vi "FID Rohwerte Linearisieren.vi"(1 "GasValue":sgl[](array[numeric]), 12 "CAL-Daten":T1={"CH4 Null"=0.0, "CH4 Steil"=[1.0, 1.0, 1.0, 1.0], "THC Null"=0.0, "THC Steil"=[1.0, 1.0, 1.0, 1.0], "NMHC Null"=0.0, "NMHC Steil"=[1.0, 1.0, 1.0, 1.0]}) -> (4 "Messwerte":sgl[](array[numeric]), 6 "Rohwert":sgl[](array[numeric]), 8 "Rohwert LIN":sgl[](array[numeric]))   [LabVIEW 2020, in "ABB-EL3000.lvlib" / "FID.lvlib" / "FID Kalibrierung.lvlib"]
uses:
  FID Kalibrierung.lvlib
  Allgemeine VI/CAL-Daten FID.ctl
  Analysator Definition/FGV Analysator Definition Aktionen.ctl
  Analysator Definition/Analysator Definition.lvlib
  Linearisierung V2/Linearisierung v2.lvlib
  FID.lvlib
  Allgemeine VI/Allgemeine VI.lvlib
panel:
  in  "Rohwert umschalten":bool
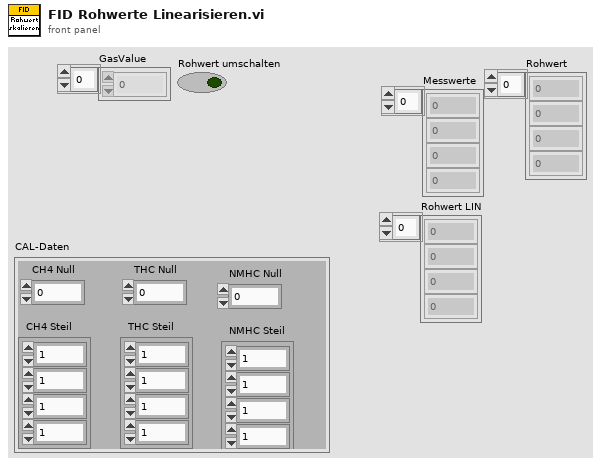
[diagram p1: front panel]
types:
  T1 = typedef "ABB-EL3000.lvlib/Allgemeine VI.lvlib/CAL-Daten FID.ctl" = cluster{"CH4 Null":sgl, "CH4 Steil":sgl[], "THC Null":sgl, "THC Steil":sgl[], "NMHC Null":sgl, "NMHC Steil":sgl[]}
  T2 = typedef "Analysator Definition.lvlib/FGV Analysator Definition Aktionen.ctl" = enum16{"lesen", "MB setzen", "MB KAL setzen", "laden"}
  T3 = typedef "Analysator Definition.lvlib/Betriebsdaten Komponente.ctl" = cluster{"Namen":string[], "MB Namen":string[], "Einheit":string, "MB Aktuell":u16, "MB Endwert":u16, "CalGase":u16[], "MB für KAL":u16[], "CG für KAL":u16[]}
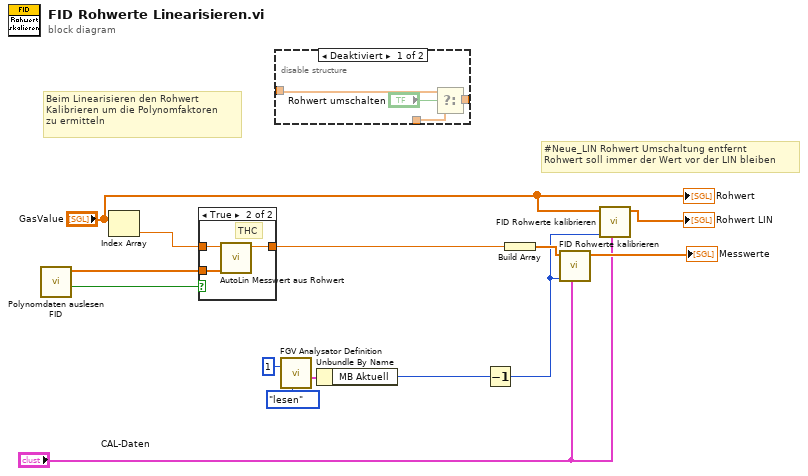
[diagram p0: block diagram]
diagram:
  # "#Neue_LIN Rohwert Umschaltung entfernt\nRohwert soll immer der Wert vor der LIN bleiben"
  # "Beim Linearisieren den Rohwert \nKalibrieren um die Polynomfaktoren \nzu ermitteln"
  n1 = call "Polynomdaten auslesen FID.vi"() -> ("Aktiv"=w5:bool, "Teil-Array"=w6:dbl[])  [unwired: 9 in, 1 out]
  n2 = Index Array(array="GasValue") -> (element=w14:sgl)  [unwired: 1 in]
  n3 = case shown="True" w5 {
    tunnel: w14 -> [w15 w18]
    tunnel: w6 -> [_ w16]
    tunnel: [w15 w17] -> w12
    frame False {
    }
    frame True {
      # "THC"
      n4 = call "AutoLin Messwert aus Rohwert.vi"("Polynomkoeff."=w16, "Rohwert (ppm)"=w18) -> ("Messwert (ppm) linearisiert"=w17:dbl)  [unwired: 9 in]
    }
  }
  n5 = disable-structure shown="Deaktiviert" {
    disable-tunnel: _ -> [w22 _]
    disable-tunnel: _ -> [w21 _]
    disable-tunnel: [w19 _] -> _
    frame Disabled {
      n6 = Select(t=w22, s="Rohwert umschalten", f=w21) -> (s? t:f=w19:dbl)
    }
    frame Enabled {
    }
  }
  n7 = call "FGV Analysator Definition.vi"("Aktionen"=FGV_Analysator_Definition_Aktionen."lesen", "Komponente"=1) -> ("Betriebsdaten Komponente"=w9:T3)  [unwired: 5 in, 4 out]
  n8 = Unbundle By Name(w9) -> ("MB Aktuell"=w7:u16)
  n9 = Decrement(x=w7) -> (x-1=w2:u16)
  n10 = Build Array(w12) -> (w13:dbl[])
  n11 = call "FID Rohwerte kalibrieren.vi"("CAL-Daten"="CAL-Daten", "Aktuelle MB"=w2, "GasValue"=w13) -> ("Kalibrierte Rohwerte"=→"Messwerte":sgl[])  [unwired: 8 in]
  n12 = call "FID Rohwerte kalibrieren.vi"("CAL-Daten"="CAL-Daten", "Aktuelle MB"=w2, "GasValue"="GasValue") -> ("Kalibrierte Rohwerte"=→"Rohwert LIN":sgl[])  [unwired: 8 in]
  "Rohwert" <- "GasValue"
